vi "3_2.vi"() -> ()   [LabVIEW 2023, in "2022.lvlib"]
uses:
  2022.lvlib
  <userlib>/_OpenG.lib/array/array.llb/Remove Duplicates from 1D Array (String)__ogtk.vi
panel:
  out "Array 3":string[](array[string])
  out "sum":i32
  out "Array 2":i32[](array[numeric])
  out "Array":string[](array[string])
  out "first subarray":string[](array[string])
  out "x+1":i32
  out "subarray":string[](array[string])
  out "array 2":string[][](array[string])
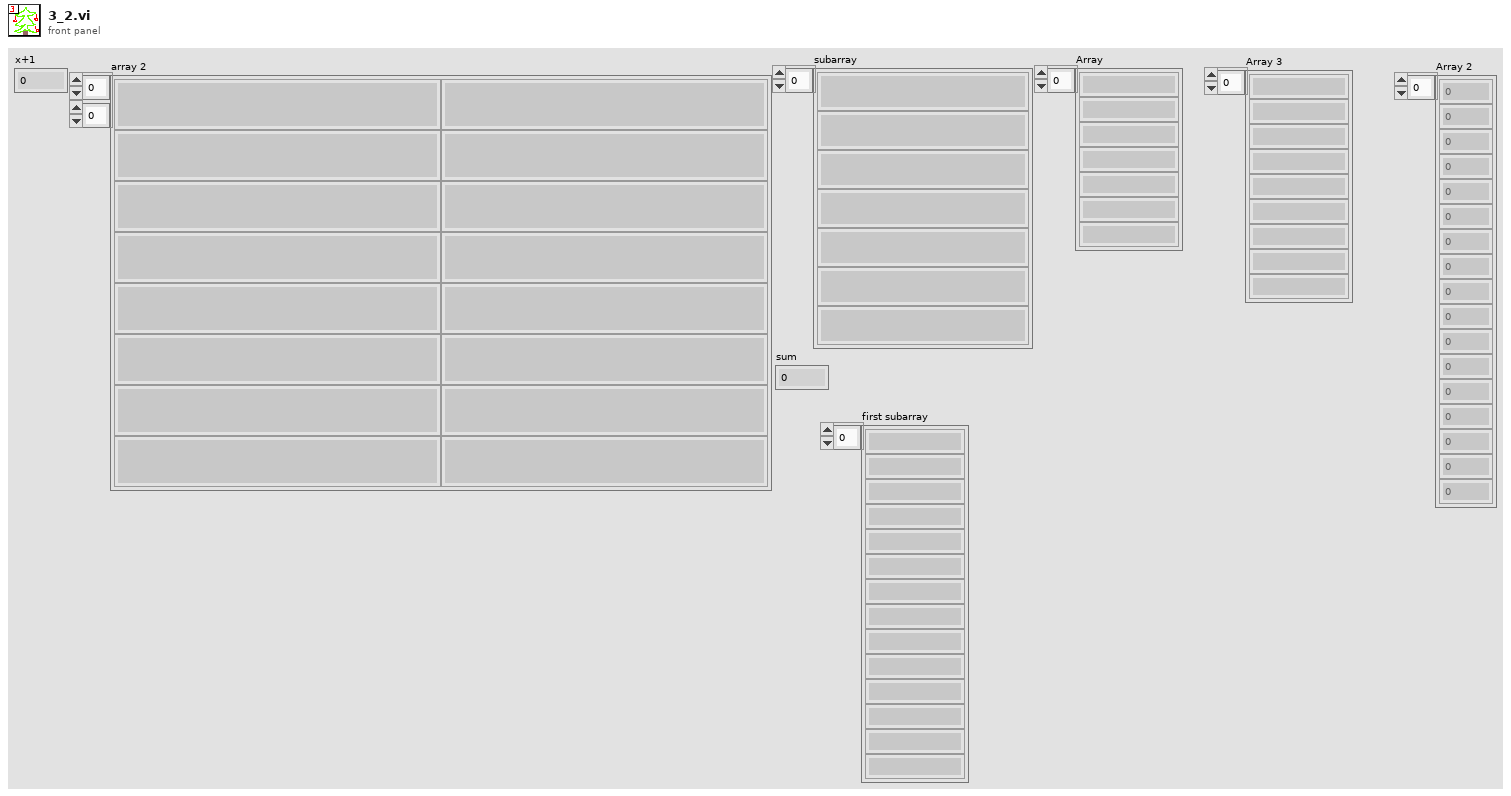
[diagram p1: front panel]
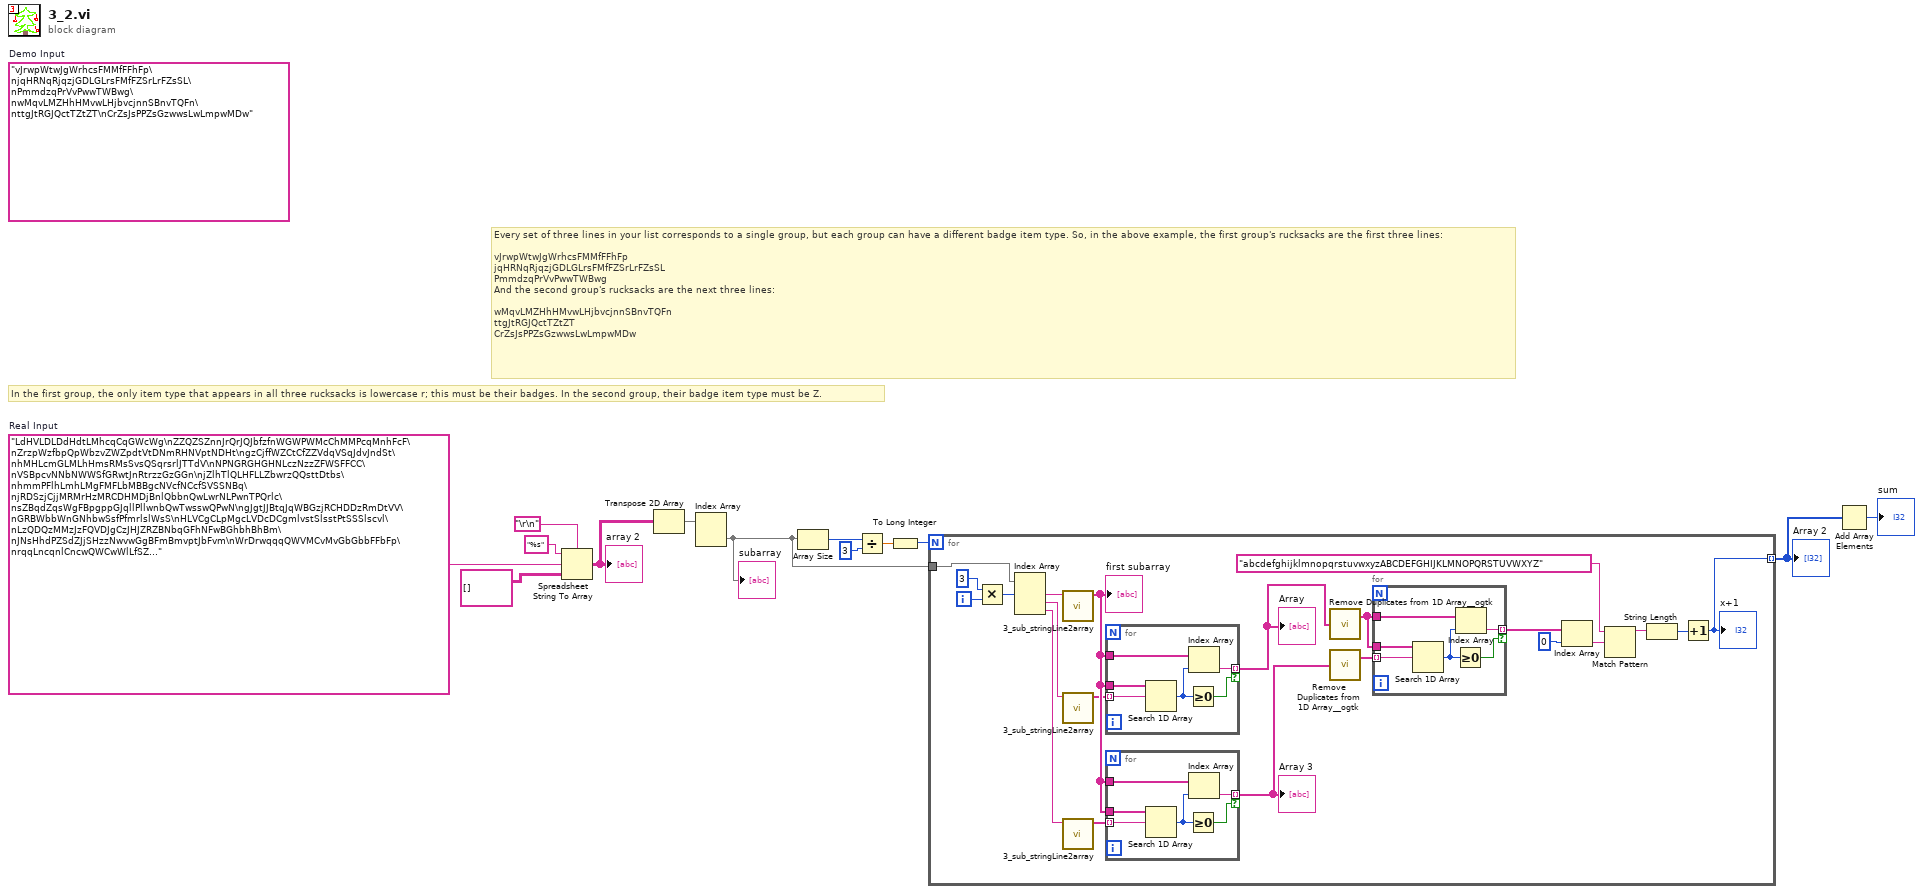
[diagram p0: block diagram]
diagram:
  w1 = "LdHVLDLDdHdtLMhcqCqGWcWg\nZZQZSZnnJrQrJQJbfzfnWGWPWMcChMMPcqMnhFcF\nZrzpWzfbpQpWbzvZWZpdtVtDNmRHNVptNDHt\ngzCjffWZCtCfZZVdqVSqJdvJndSt\nhMHLcmGLMLhHmsRMsSvsQSqrsrlJTTdV\nNPNGRGHGHNLczNzzZFWSFFCC\nVSBpcvNNbNWWSfGRwtJnRtrzzGzGGn\njZlhTlQLHFLLZbwrzQQsttDtbs\nhmmPFlhLmhLMgFMFLbMBBgcNVcfNCcfSVSSNBq\njRDSzjCjjMRMrHzMRCDHMDjBnlQbbnQwLwrNLPwnTPQrlc\nsZBqdZqsWgFBpgppGJqllPllwnbQwTwsswQPwN\ngJgtJJBtqJqWBGzjRCHDDzRmDtVV\nGRBWbbWnGNhbwSsfPfmrlslWsS\nHLVCgCLpMgcLVDcDCgmlvstSlsstPtSSSlscvl\nLzQDQzMMzJzFQVDJgCzJHJZRZBNbqGFhNFwBGhbhBhBm\nJNsHhdPZSdZJjSHzzNwvwGgBFmBmvptJbFvm\nWrDrwqqqQWVMCvMvGbGbbFFbFp\nrqqLncqnlCncwQWCwWlLfSZ..."  # Real Input
  (unwired) "vJrwpWtwJgWrhcsFMMfFFhFp\njqHRNqRjqzjGDLGLrsFMfFZSrLrFZsSL\nPmmdzqPrVvPwwTWBwg\nwMqvLMZHhHMvwLHjbvcjnnSBnvTQFn\nttgJtRGJQctTZtZT\nCrZsJsPPZsGzwwsLwLmpwMDw"  # Demo Input
  # "In the first group, the only item type that appears in all three rucksacks is lowercase r; this must be their badges. In the second group, their badge item type must be Z."
  # "Every set of three lines in your list corresponds to a single group, but each group can have a different badge item type. So, in the above example, the first group's rucksacks are the first three lines:\n\nvJrwpWtwJgWrhcsFMMfFFhFp\njqHRNqRjqzjGDLGLrsFMfFZSrLrFZsSL\nPmmdzqPrVvPwwTWBwg\nAnd the second group's rucksacks are the next three lines:\n\nwMqvLMZHhHMvwLHjbvcjnnSBnvTQFn\nttgJtRGJQctTZtZT\nCrZsJsPPZsGzwwsLwLmpwMDw"
  n1 = Spreadsheet String To Array(delimiter (Tab)="\r\n", format string="%s", spreadsheet string=w1, array type (2D Dbl)=string[][] []) -> (array=w10:string[][])
  "array 2" <- w10
  n2 = Transpose 2D Array(2D array=w10) -> (transposed array=w9:string[][])
  n3 = Index Array(array=w9) -> (element=w6:string[])  [unwired: 2 in]
  "subarray" <- w6
  n4 = Array Size(array=w6) -> (size(s)=w5:i32)
  n5 = Divide(x=w5, y=3) -> (x/y=w4:dbl)
  n6 = To Long Integer(number=w4) -> (32bit integer=w2:i32)
  n7 = for {
    N: w2 -> [_]
    tunnel: [w30] -> w8 mode=indexing
    tunnel: w6 -> [w28]
    i -> [w27]
    n8 = Multiply(x=3, y=w27) -> (x*y=w25:i32)
    n9 = Index Array(array=w28, index #1=w25) -> (element #1=w24:string, element #2=w23:string, element #3=w22:string)  [unwired: 2 in]
    n10 = call "3_sub_stringLine2array.vi"("String"=w24) -> ("Array"=w21:string[])  [unwired: 10 in]
    "first subarray" <- w21
    n11 = call "3_sub_stringLine2array.vi"("String"=w23) -> ("Array"=w20:string[])  [unwired: 10 in]
    n12 = call "3_sub_stringLine2array.vi"("String"=w22) -> ("Array"=w19:string[])  [unwired: 10 in]
    n13 = for {
      tunnel: w21 -> [w50]
      tunnel: w21 -> [w52]
      tunnel: [w48] -> w18 mode=indexing if=w51
      tunnel: w20 -> [w47] mode=indexing
      n14 = Search 1D Array(1D array=w52, element=w47) -> (index of element=w49:i32)  [unwired: 1 in]
      n15 = Greater Or Equal To 0?(x=w49) -> (x >= 0?=w51:bool)
      n16 = Index Array(array=w50, index=w49) -> (element=w48:string)
    }
    "Array" <- w18
    n17 = for {
      tunnel: w21 -> [w44]
      tunnel: w21 -> [w46]
      tunnel: [w42] -> w17 mode=indexing if=w45
      tunnel: w19 -> [w41] mode=indexing
      n18 = Search 1D Array(1D array=w46, element=w41) -> (index of element=w43:i32)  [unwired: 1 in]
      n19 = Greater Or Equal To 0?(x=w43) -> (x >= 0?=w45:bool)
      n20 = Index Array(array=w44, index=w43) -> (element=w42:string)
    }
    "Array 3" <- w17
    n21 = call-poly <userlib>:"Remove Duplicates from 1D Array__ogtk.vi"("Input Array"=w18) -> ("Output Array"=w16:string[])  [unwired: 1 out]
    n22 = call-poly <userlib>:"Remove Duplicates from 1D Array__ogtk.vi"("Input Array"=w17) -> ("Output Array"=w15:string[])  [unwired: 1 out]
    n23 = for {
      tunnel: w16 -> [w38]
      tunnel: w16 -> [w40]
      tunnel: [w36] -> w14 mode=indexing if=w39
      tunnel: w15 -> [w35] mode=indexing
      n24 = Search 1D Array(1D array=w40, element=w35) -> (index of element=w37:i32)  [unwired: 1 in]
      n25 = Greater Or Equal To 0?(x=w37) -> (x >= 0?=w39:bool)
      n26 = Index Array(array=w38, index=w37) -> (element=w36:string)
    }
    n27 = Index Array(array=w14, index=0) -> (element=w29:string)
    n28 = Match Pattern(string="abcdefghijklmnopqrstuvwxyzABCDEFGHIJKLMNOPQRSTUVWXYZ" ("y"), regular expression=w29) -> (before substring=w33:string)  [unwired: 1 in, 3 out]
    n29 = String Length(string=w33) -> (length=w34:i32)
    n30 = Increment(x=w34) -> (x+1=w30:i32)
    "x+1" <- w30
  }
  "Array 2" <- w8
  n31 = Add Array Elements(numeric array=w8) -> (sum=→"sum":i32)
